vi "Read Payload.vi"(4 "MaskingKey":u8[](array[numeric]), 6 "Mask":bool, 8 "error in (no error)":errorcluster, 9 "Timeout ms":i32, 10 "Count":u64, 11 "WebSocket Client in":refnum<class "WebSocket Client.lvclass">) -> (0 "error out":errorcluster, 1 "Remaining  Timeout":i32, 2 "Payload":string, 3 "WebSocket Client out":refnum<class "WebSocket Client.lvclass">)   [LabVIEW 2020, in "HTTP Server.lvlib" / "WebSocket Client.lvclass"]
uses:
  WebSocket Client.lvclass
  WebSocket Client.lvclass/WebSocket Client.ctl
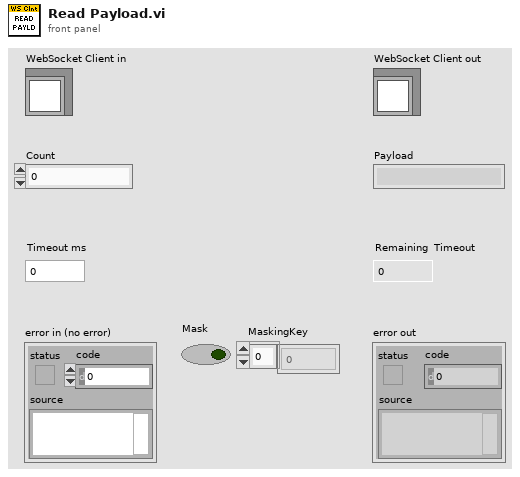
[diagram p1: front panel]
types:
  T1 = enum16{"Standard", "Buffered", "CRLF", "Immediate"}
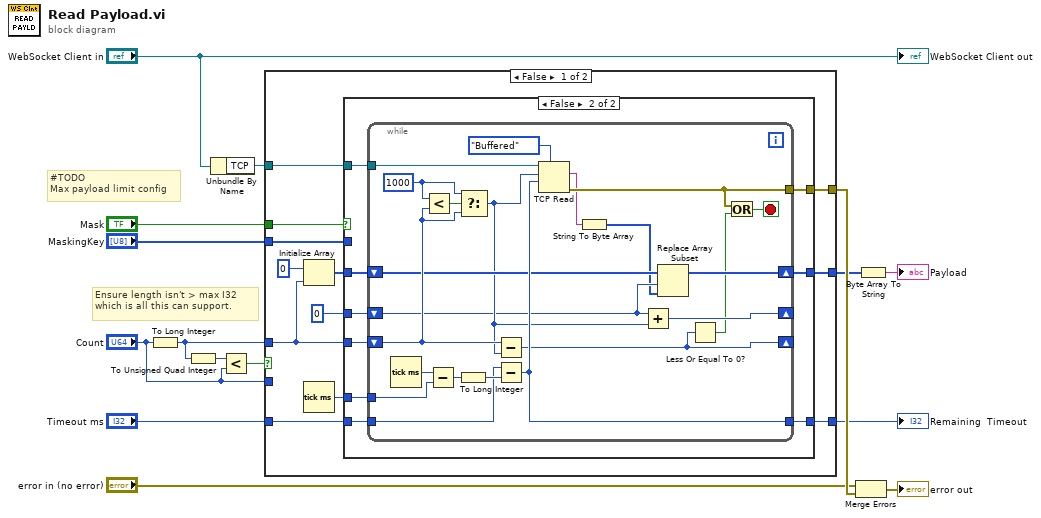
[diagram p0: block diagram]
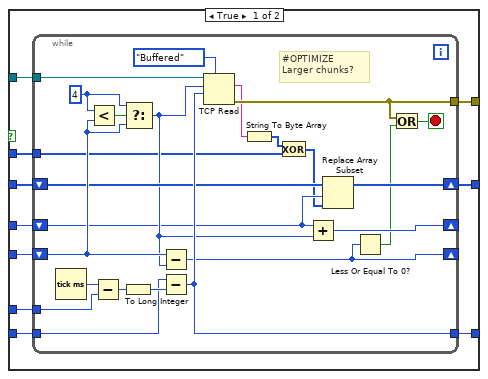
[diagram p2: hidden frame]
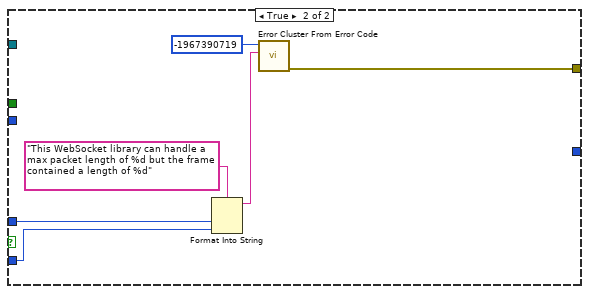
[diagram p3: hidden frame]
diagram:
  # "#TODO\nMax payload limit config"
  # "Ensure length isn't > max I32 which is all this can support."
  n1 = To Long Integer(number="Count") -> (32bit integer=w12:i32)
  n2 = To Unsigned Quad Integer(1:w12) -> (0:w14:u64)
  n3 = Unbundle By Name("WebSocket Client in") -> ("TCP"=w8:refnum<k5>)
  n4 = Less?(x=w14, y="Count") -> (x < y?=w13:bool)
  n5 = case shown="False" w13 {
    tunnel: [w16 w95] -> w15
    tunnel: w12 -> [w19 w94]
    tunnel: "Mask" -> [w26 _]
    tunnel: "MaskingKey" -> [w25 _]
    tunnel: "Timeout ms" -> [w24 _]
    tunnel: "Count" -> [_ w93]
    tunnel: [w21 _] -> w1
    tunnel: w8 -> [w20 _]
    tunnel: [w17 _] -> w7
    frame False {
      n6 = Initialize Array(u8 0, w19) -> (w23:u8[])
      n7 = Tick Count (ms)() -> (millisecond timer value=w22:u32)
      n8 = case shown="False" w26 {
        tunnel: w25 -> [w30 _]
        tunnel: w24 -> [w35 w68]
        tunnel: w23 -> [w37 w70]
        tunnel: w22 -> [w36 w69]
        tunnel: [w34 w67] -> w21
        tunnel: w20 -> [w33 w66]
        tunnel: w19 -> [w32 w65]
        tunnel: 0 -> [w31 w64]
        tunnel: [w29 w63] -> w17
        tunnel: [w28 w62] -> w16
        frame True {
          n9 = while {
            shift-right: [w45] -> w29
            shift-left: w37 -> [w49]
            tunnel: w36 -> [w60]
            tunnel: w35 -> [w57]
            tunnel: [w55] -> w34
            tunnel: w33 -> [w56]
            shift-right: [w44] -> _
            shift-left: w32 -> [w50]
            shift-right: [w47] -> _
            shift-left: w31 -> [w40]
            tunnel: w30 -> [w46]
            tunnel: [w41] -> w28
            stop <- w42 stop-if-true
            w53 = 4
            # "#OPTIMIZE\nLarger chunks?"
            n10 = Tick Count (ms)() -> (millisecond timer value=w61:u32)
            n11 = Less?(x=w53, y=w50) -> (x < y?=w54:bool)
            n12 = Subtract(x=w61, y=w60) -> (x-y=w59:u32)
            n13 = To Long Integer(number=w59) -> (32bit integer=w58:i32)
            n14 = Select(t=w53, s=w54, f=w50) -> (s? t:f=w48:i32)
            n15 = Subtract(x=w50, y=w48) -> (x-y=w44:i32)
            n16 = Subtract(x=w57, y=w58) -> (x-y=w55:i32)
            n17 = TCP Read(connection ID=w56, bytes to read=w48, 7:T1."Buffered" ("mode (standard)"), 9:w55) -> (data out=w38:string, error out=w41:errorcluster)  [unwired: 1 in, 1 out]
            n18 = String To Byte Array(string=w38) -> (unsigned byte array=w51:u8[])
            n19 = Exclusive Or(1:w46, 2:w51) -> (0:w39:u8[])
            n20 = Add(x=w40, y=w48) -> (x+y=w47:i32)
            n21 = Replace Array Subset(array=w49, new element=w39, index=w40) -> (w45:u8[])
            n22 = Less Or Equal To 0?(x=w44) -> (x <= 0?=w43:bool)
            n23 = Or(x=w41, y=w43) -> (x .or. y?=w42:bool)
          }
        }
        frame False {
          n24 = while {
            shift-right: [w76] -> w63
            shift-left: w70 -> [w79]
            tunnel: w69 -> [w90]
            tunnel: w68 -> [w87]
            tunnel: [w85] -> w67
            tunnel: w66 -> [w86]
            shift-right: [w75] -> _
            shift-left: w65 -> [w80]
            shift-right: [w77] -> _
            shift-left: w64 -> [w72]
            tunnel: [w92] -> w62
            stop <- w73 stop-if-true
            w83 = 1000
            n25 = Tick Count (ms)() -> (millisecond timer value=w91:u32)
            n26 = Less?(x=w83, y=w80) -> (x < y?=w84:bool)
            n27 = Subtract(x=w91, y=w90) -> (x-y=w89:u32)
            n28 = To Long Integer(number=w89) -> (32bit integer=w88:i32)
            n29 = Select(t=w83, s=w84, f=w80) -> (s? t:f=w78:i32)
            n30 = Subtract(x=w80, y=w78) -> (x-y=w75:i32)
            n31 = Subtract(x=w87, y=w88) -> (x-y=w85:i32)
            n32 = TCP Read(connection ID=w86, bytes to read=w78, 7:T1."Buffered" ("mode (standard)"), 9:w85) -> (data out=w81:string, error out=w92:errorcluster)  [unwired: 1 in, 1 out]
            n33 = String To Byte Array(string=w81) -> (unsigned byte array=w71:u8[])
            n34 = Add(x=w72, y=w78) -> (x+y=w77:i32)
            n35 = Replace Array Subset(array=w79, new element=w71, index=w72) -> (w76:u8[])
            n36 = Less Or Equal To 0?(x=w75) -> (x <= 0?=w74:bool)
            n37 = Or(x=w92, y=w74) -> (x .or. y?=w73:bool)
          }
        }
      }
    }
    frame True {
      n38 = Format Into String(format string="This WebSocket library can handle a max packet length of %d but the frame contained a length of %d" ("error message (\"\")"), w94, w93) -> (resulting string=w96:string)  [unwired: 2 in, 1 out]
      n39 = call <vilib>:"Error Cluster From Error Code.vi"("error message (\"\")"=w96, "error code (0)"=-1967390719) -> ("error out"=w95:errorcluster)  [unwired: 7 in]
    }
  }
  "Remaining  Timeout" <- w1
  n40 = Merge Errors("error in (no error)", w15) -> (→"error out":errorcluster)
  n41 = Byte Array To String(unsigned byte array=w7) -> (string=→"Payload":string)
  "WebSocket Client out" <- "WebSocket Client in"
